vi "LuaVIEW Console.vi"(1 "print string":string) -> ()   [LabVIEW 2012]
panel:
  out "console":string
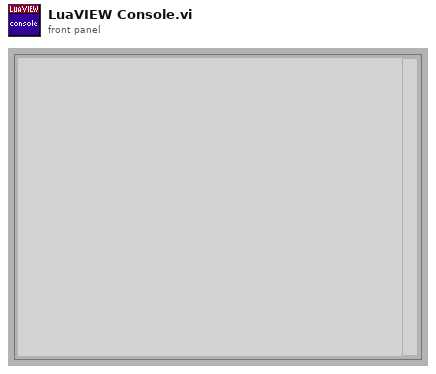
[diagram p1: front panel]
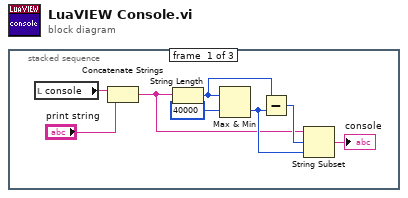
[diagram p0: block diagram]
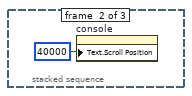
[diagram p2: hidden frame]
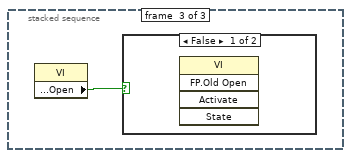
[diagram p3: hidden frame]
diagram:
  n1 = stacked-sequence {
    frame #0 {
      n2 = local read "console"() -> (w8:string)
      n3 = Concatenate Strings(w8, "print string") -> (w2:string)
      n4 = String Length(string=w2) -> (length=w6:i32)
      n5 = Max & Min(x=w6, y=40000) -> (min(x,y)=w5:i32)  [unwired: 1 out]
      n6 = Subtract(x=w6, y=w5) -> (x-y=w4:i32)
      n7 = String Subset(string=w2, offset (0)=w4, length (rest)=w5) -> (substring=→"console":string)
    }
    frame #1 {
      n8 = property on="console" class="Str"("Text.Scroll Position"=u32 40000) -> ()  [unwired: 2 in, 2 out]
    }
    frame #2 {
      n9 = property class="VI"() -> ("Front Panel Window:Open"=w10:bool)  [unwired: 2 in, 2 out]
      n10 = case shown="False" w10 {
        frame False {
          n11 = invoke class="VI" method="FP.Old Open"() -> ()  [unwired: 5 in, 5 out]
        }
        frame True {
        }
      }
    }
  }
